vi "Pose2D_msg.vi"(11 "Reply":string) -> (3 "输出簇":cluster{"rot_z":dbl, "lin_x":dbl})   [LabVIEW 2014]
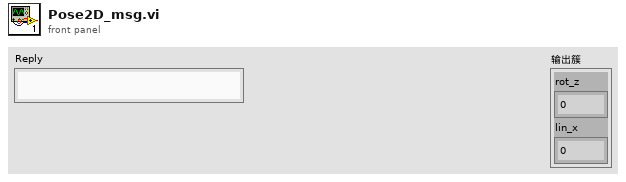
[diagram p1: front panel]
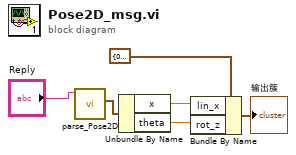
[diagram p0: block diagram]
diagram:
  n1 = call <vilib>:"parse_Pose2D.vi"("msg in"="Reply") -> ("Pose 2D"=w4:cluster{"x":dbl, "y":dbl, "theta":dbl})  [unwired: 4 in, 2 out]
  n2 = Unbundle By Name(w4) -> ("x"=w3:dbl, "theta"=w2:dbl)
  n3 = Bundle By Name(cluster=cluster{"rot_z":dbl, "lin_x":dbl} {"rot_z"=0.0, "lin_x"=0.0} ("vel_cal"), "lin_x"=w3, "rot_z"=w2) -> (→"输出簇":cluster{"rot_z":dbl, "lin_x":dbl})
